vi "Data.vi"(11 "Set Error Msg in":refnum<class "Set Error Msg.lvclass">) -> (1 "Override":errorcluster, 2 "Merge":errorcluster)   [LabVIEW 2021, in "Set Error.lvlib" / "Set Error Msg.lvclass"]
uses:
  Set Error Msg.lvclass
  Set Error Msg.lvclass/Set Error Msg.ctl
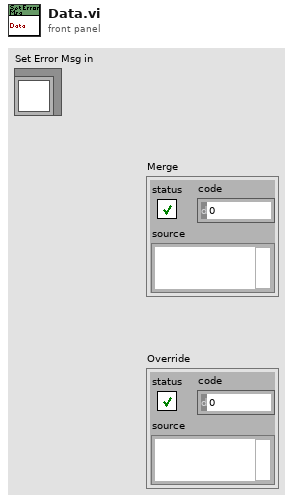
[diagram p1: front panel]
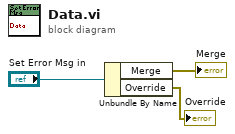
[diagram p0: block diagram]
diagram:
  n1 = Unbundle By Name("Set Error Msg in") -> ("Merge"=→"Merge":errorcluster, "Override"=→"Override":errorcluster)
